vi "Split.vi"(6 "Groups":string[][](array[string]), 8 "error in (no error)":errorcluster caption="entrée d'erreur (pas d'erreur)", 9 "y":string[][](array[string]), 10 "X":string[][](array[string]), 11 "TimeSeriesSplit.lvclass":refnum<class "TimeSeriesSplit.lvclass">) -> (0 "error out":errorcluster caption="sortie d'erreur", 2 "Split":T1(array[cluster]), 3 "TimeSeriesSplit.lvclass":refnum<class "TimeSeriesSplit.lvclass">)   [LabVIEW 2020, in "TimeSeriesSplit.lvclass"]
doc: "Returns :\n\n- train : ndarray\n The training set indices for that split.\n\n- test : ndarray\n The testing set indices for that split."
uses:
  TimeSeriesSplit.lvclass
  TimeSeriesSplit.lvclass/TimeSeriesSplit.ctl
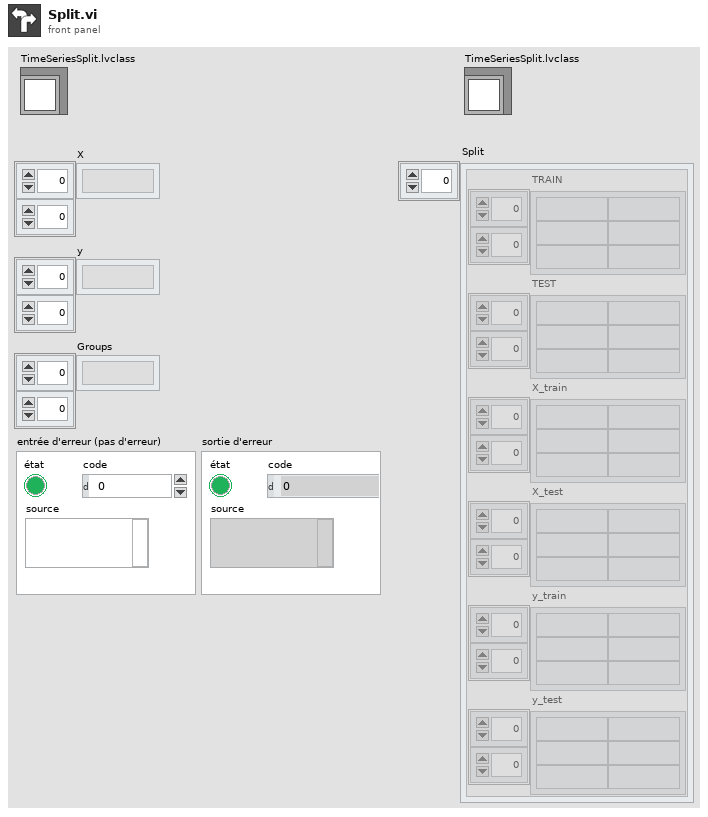
[diagram p1: front panel]
types:
  T1 = cluster{"TRAIN":string[][], "TEST":string[][], "X_train":string[][], "X_test":string[][], "y_train":string[][], "y_test":string[][]}[]
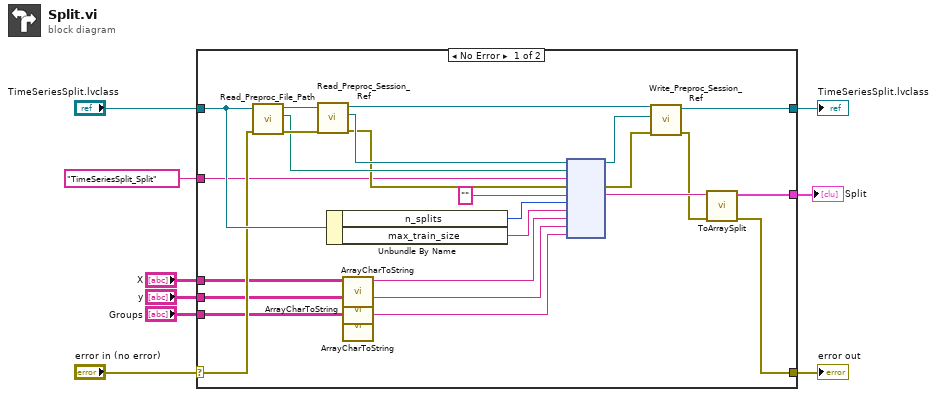
[diagram p0: block diagram]
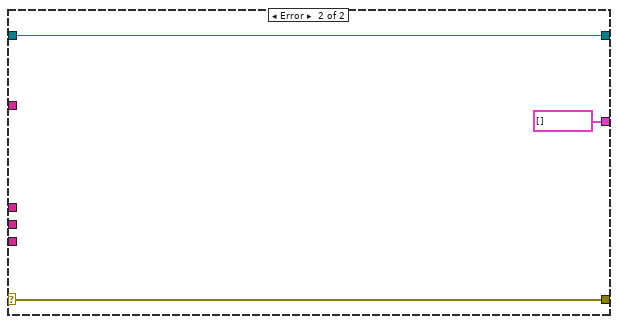
[diagram p2: hidden frame]
diagram:
  n1 = case shown="No Error" "error in (no error)" {
    selector: "error in (no error)" -> [w24 w37]
    tunnel: [w11 w37] -> w8
    tunnel: [w14 w36] -> w6
    tunnel: "TimeSeriesSplit.lvclass" -> [w25 w36]
    tunnel: "TimeSeriesSplit_Split" -> [w23 _]
    tunnel: "X" -> [w20 _]
    tunnel: "y" -> [w19 _]
    tunnel: "Groups" -> [w18 _]
    tunnel: [w10 T1 [] ("Split")] -> w1
    frame No Error {
      n2 = call-dynamic "Read_Preproc_File_Path.vi"("error in (no error)"=w24, "Python in"=w25) -> ("error out"=w33:errorcluster, "File_Path"=w32:path, "Python out"=w34:refnum<class "TimeSeriesSplit.lvclass">)  [unwired: 7 in]
      n3 = call-dynamic "Read_Preproc_Session_Ref.vi"("error in (no error)"=w33, "Python in"=w34) -> ("error out"=w30:errorcluster, "Session_ref"=w31:refnum<k35>, "Python out"=w29:refnum<class "TimeSeriesSplit.lvclass">)  [unwired: 7 in]
      n4 = Unbundle By Name(w25) -> ("n_splits"=w22:i32, "max_train_size"=w21:string)
      n5 = call "ArrayCharToString.vi"("TAB"=w20) -> ("Instruction"=w17:string)  [unwired: 10 in]
      n6 = call "ArrayCharToString.vi"("TAB"=w19) -> ("Instruction"=w16:string)  [unwired: 10 in]
      n7 = call "ArrayCharToString.vi"("TAB"=w18) -> ("Instruction"=w15:string)  [unwired: 10 in]
      n8 = node(w31, w32, w23, w30, "", w22, w21, w17, w16, w15) -> (w27:refnum<k35>, w28:errorcluster, w13:string)  [unwired: 5 in, 2 out]
      n9 = call-dynamic "Write_Preproc_Session_Ref.vi"("error in (no error)"=w28, "Session_ref"=w27, "Python in"=w29) -> ("error out"=w12:errorcluster, "Python out"=w14:refnum<class "TimeSeriesSplit.lvclass">)  [unwired: 7 in]
      n10 = call "ToArraySplit.vi"("sortie d'erreur"=w12, "Return value"=w13) -> ("sortie d'erreur"=w11:errorcluster, "Split"=w10:T1)  [unwired: 8 in]
    }
    frame Error {
    }
  }
  "error out" <- w8
  "TimeSeriesSplit.lvclass" <- w6
  "Split" <- w1
